vi "Equi-Ripple BandStop (CDB).vi"(0 "X":cdb[](array[numeric]), 1 "lower pass freq":dbl=0.2 format="%0.2f", 3 "# of taps":i32=33, 4 "lower stop freq":dbl=0.25000000000000006 format="%0.2f", 5 "higher pass freq":dbl=0.4000000000000001 format="%0.2f", 8 "higher stop freq":dbl=0.3500000000000001 format="%0.2f", 9 "sampling freq: fs":dbl=1.0 format="%0.2f") -> (6 "Filtered X":cdb[](array[numeric]), 7 "error":i32)   [LabVIEW 2018, in "NI_AALBase.lvlib"]
doc: "Generates a bandstop FIR digital filter with equi-ripple characteristics using the Parks-McClellan algorithm and <B>higher pass freq</B>, <B>lower pass freq</B>, <B># of taps</B>, <B>lower stop freq</B>, <B>higher stop freq</B>, and <B>sampling freq: fs</B>. The Equi-Ripple BandStop VI then applies a linear-phase, bandstop filter to the input sequence <B>X</B> using the Convolution VI to obtain <B>Filtered X</B>. Wire data to the <B>X</B> input to determine the polymorphic instance to use or manually select the instance."
uses:
  NI_AALBase.lvlib
  1D Convolution (DBL).vi
  NI_AALPro.lvlib
panel:
  # "Equi-Ripple\n BandStop FIR Filter"
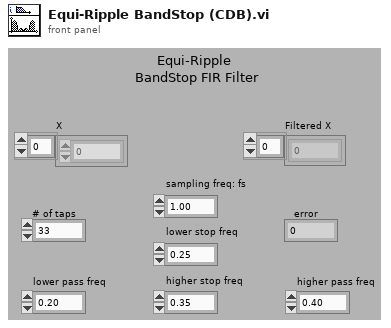
[diagram p1: front panel]
types:
  T1 = cluster{"Amplitude":dbl, "DC":dbl, "lower pass freq":dbl, "Weight":dbl}
  T2 = cluster{"Amplitude":dbl, "lower stop freq":dbl, "higher stop freq":dbl, "Weight":dbl}
  T3 = cluster{"Amplitude":dbl, "higher pass freq":dbl, dbl, "Weight":dbl}
  T4 = cluster{"Amplitude":dbl, "higher pass freq":dbl, "higher stop freq":dbl, "Weight":dbl}[]
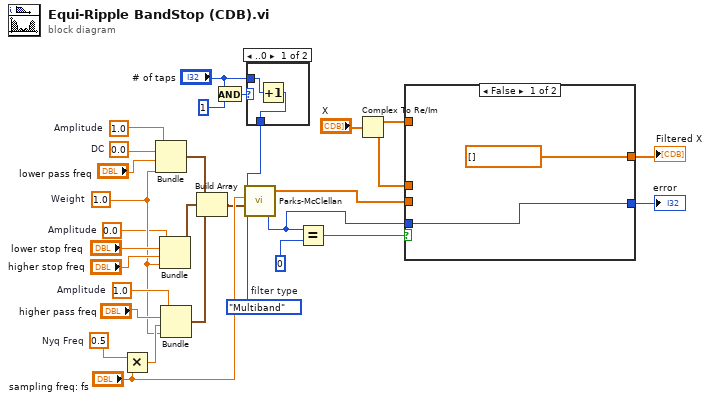
[diagram p0: block diagram]
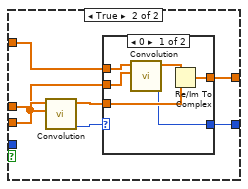
[diagram p2: hidden frame]
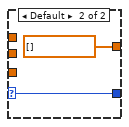
[diagram p3: hidden frame]
diagram:
  w15 = enum32{"Multiband", "Differentiator", "Hilbert"}."Multiband"  # filter type
  w13 = 1.0  # Amplitude
  w28 = 0.5  # Nyq Freq
  w11 = 0.0  # Amplitude
  w12 = 1.0  # Weight
  w10 = 0.0  # DC
  w9 = 1.0  # Amplitude
  n1 = Multiply(x=w28, y="sampling freq: fs") -> (x*y=w20:dbl)
  n2 = Bundle("Amplitude"=w9, "DC"=w10, "lower pass freq"="lower pass freq", "Weight"=w12) -> (w27:T1)  [unwired: 1 in]
  n3 = Bundle("Amplitude"=w11, "lower stop freq"="lower stop freq", "higher stop freq"="higher stop freq", "Weight"=w12) -> (w26:T2)  [unwired: 1 in]
  n4 = Bundle("Amplitude"=w13, "higher pass freq"="higher pass freq", w20, "Weight"=w12) -> (w19:T3)  [unwired: 1 in]
  n5 = Build Array(w27, w26, w19) -> (w16:T4)
  n6 = And(x="# of taps", y=1) -> (x .and. y?=w24:i32)
  n7 = case shown="..0" w24 {
    tunnel: "# of taps" -> [w32 w33]
    tunnel: [w31 w33] -> w18
    frame ..0 {
      n8 = Increment(x=w32) -> (x+1=w31:i32)
    }
    frame 1.. {
    }
  }
  n9 = call "Parks-McClellan.vi"("filter type"=w15, "Band Parameters"=w16, "sampling freq: fs"="sampling freq: fs", "# of taps"=w18) -> ("error"=w7:i32, "h"=w8:dbl[])  [unwired: 1 out]
  n10 = Equal?(x=w7, y=0) -> (x = y?=w6:bool)
  n11 = Complex To Re/Im(x + iy="X") -> (x=w4:dbl[], y=w3:dbl[])
  n12 = case shown="False" w6 {
    tunnel: w7 -> [w35 _]
    tunnel: [w35 w36] -> w1
    tunnel: [cdb[] [] ("empty array") w38] -> w2
    tunnel: w3 -> [_ w42]
    tunnel: w8 -> [_ w39]
    tunnel: w4 -> [_ w40]
    frame False {
    }
    frame True {
      n13 = call-poly "Convolution.vi"("Y"=w39, "X"=w42) -> ("error"=w41:i32, "X * Y"=w37:dbl[])  [unwired: 8 in]
      n14 = case shown="0" w41 {
        selector: w41 -> [_ w49]
        tunnel: w40 -> [w48 _]
        tunnel: w39 -> [w47 _]
        tunnel: [w45 cdb[] [] ("empty array")] -> w38
        tunnel: w37 -> [w46 _]
        tunnel: [w44 w49] -> w36
        frame 0 {
          n15 = call-poly "Convolution.vi"("Y"=w47, "X"=w48) -> ("error"=w44:i32, "X * Y"=w43:dbl[])  [unwired: 8 in]
          n16 = Re/Im To Complex(1:w46, 2:w43) -> (0:w45:cdb[])
        }
        frame Default {
        }
      }
    }
  }
  "Filtered X" <- w2
  "error" <- w1
